vi "Read Data.vi"(8 "error in (no error)":errorcluster, 11 "Tool Dots in":refnum<class "Tool Dots.lvclass">) -> (0 "error out":errorcluster, 2 "Dot.lvclass":refnum<class "Dot.lvclass">, 3 "Tool Dots out":refnum<class "Tool Dots.lvclass">)   [LabVIEW 2019, in "Tool Dots.lvclass"]
uses:
  Tool Dots.lvclass
  Parse/Dot/Dot.lvclass
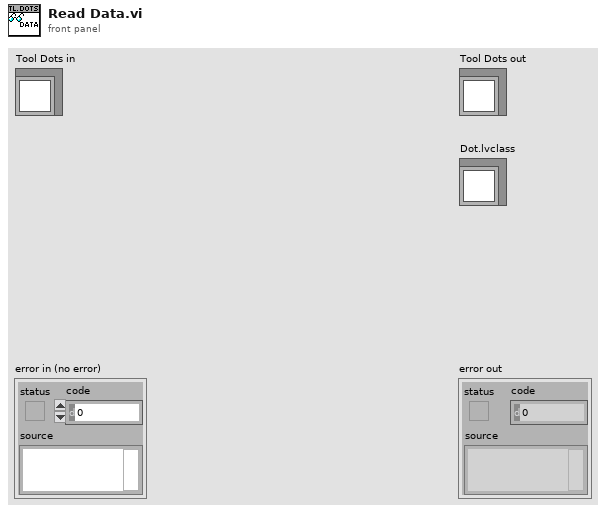
[diagram p1: front panel]
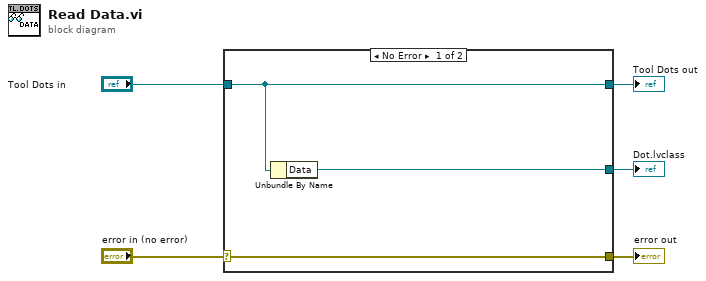
[diagram p0: block diagram]
diagram:
  n1 = case shown="No Error" "error in (no error)" {
    selector: "error in (no error)" -> [w8 w9]
    tunnel: [w8 w9] -> w4
    tunnel: [w7 w10] -> w2
    tunnel: "Tool Dots in" -> [w7 w10]
    tunnel: [w6 _] -> w1
    frame No Error {
      n2 = Unbundle By Name(w7) -> ("Data"=w6:refnum<class "Dot.lvclass">)
    }
    frame Error {
    }
  }
  "error out" <- w4
  "Tool Dots out" <- w2
  "Dot.lvclass" <- w1
